vi "PythonWrapper.vi"(4 "PythonPath":path, 6 "PythonVersion":string, 7 "SessionName":string, 8 "error in (no error)":errorcluster, 11 "ModulePath":path) -> (0 "error out":errorcluster, 3 "PythonWrapper":refnum<class "PythonWrapper.lvclass">)   [LabVIEW 2022 SP3, in "PythonWrapper.lvlib" / "PythonWrapper.lvclass"]
uses:
  PythonWrapper.lvclass
  C:/Users/jakub/repos/gh/sw4sys/lv-python-wrapper/PythonWrapper/Source/PythonSession/PythonSession.lvclass
  PythonSession/PythonSession.lvclass/PythonSession.ctl
  PythonWrapper.lvclass/PythonWrapper.ctl
  PythonSession/Write SessionName.vi
  PythonSession/Write PythonVersion.vi
  PythonSession/Write PythonPath.vi
  Write ModulePath.vi
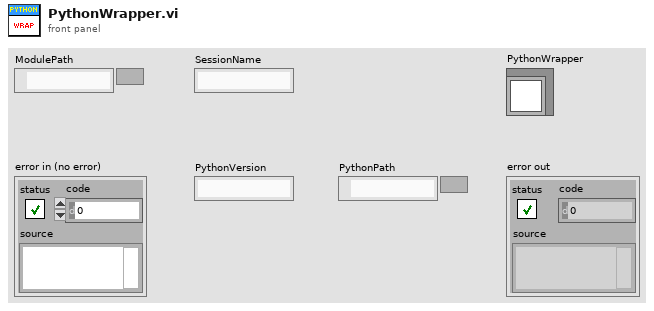
[diagram p1: front panel]
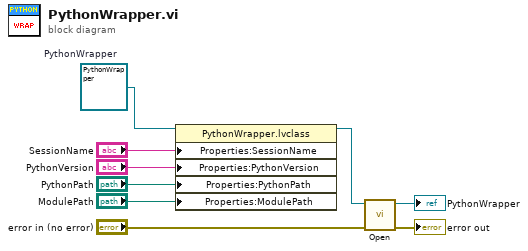
[diagram p0: block diagram]
diagram:
  w5 = refnum<class "PythonWrapper.lvclass"> refnum  # PythonWrapper
  n1 = property class="PythonWrapper.lvclass"(reference=w5, "Properties:SessionName"="SessionName", "Properties:PythonVersion"="PythonVersion", "Properties:PythonPath"="PythonPath", "Properties:ModulePath"="ModulePath") -> (reference out=w6:refnum<class "PythonWrapper.lvclass">)  [unwired: 1 in, 1 out]
  n2 = call-dynamic "Open.vi"("error in (no error)"="error in (no error)", "PythonWrapper in"=w6) -> ("error out"=→"error out":errorcluster, "PythonWrapper out"=→"PythonWrapper":refnum<class "PythonWrapper.lvclass">)  [unwired: 8 in]
